vi "fpgaLED.vi"(7 "FPGA I/O In":refnum<k21>="IO Module\\D0 0", 8 "Testpulse Time Delay (20 ns ticks)":u32=15, 9 "Testpulse Separation (20 ns ticks)":u32=500, 10 "Testpulse duration (20 ns ticks)":u32=1, 11 "Testpulser On/Off":bool) -> (0 "Total number of pulses sent":u64, 3 "Is Test Pulse?":bool)   [LabVIEW 2012]
uses:
  <vilib>/rvi/eio/common/nirviEmuTemplateMethod_errors.vi
  <vilib>/eio/EIONode/EIONode.xnode
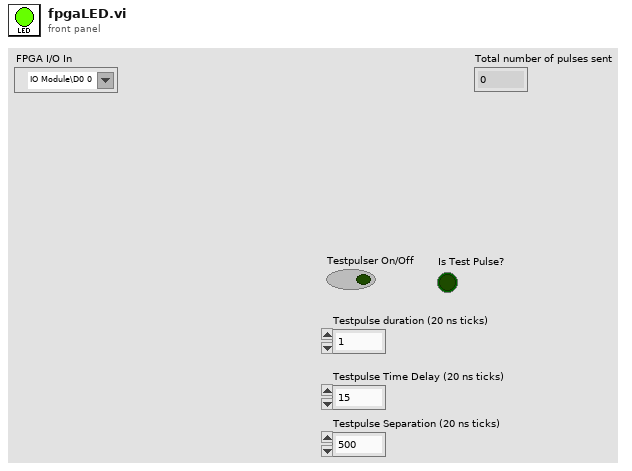
[diagram p1: front panel]
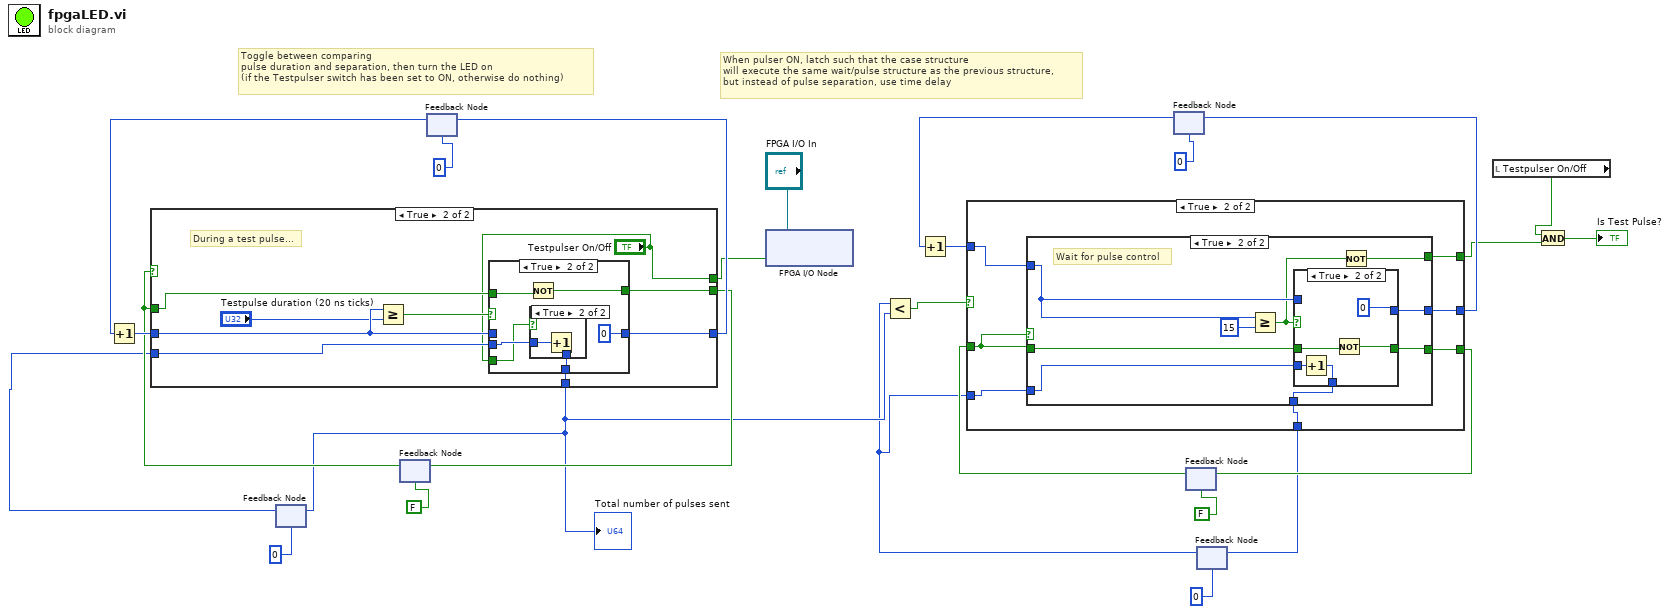
[diagram p0: block diagram]
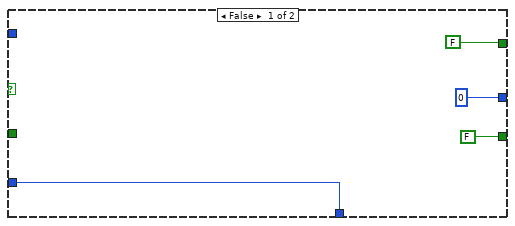
[diagram p2: hidden frame]
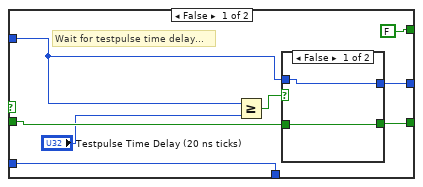
[diagram p3: hidden frame]
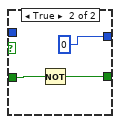
[diagram p4: hidden frame]
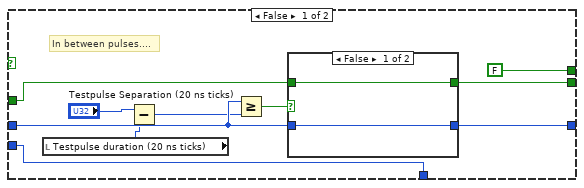
[diagram p6: hidden frame]
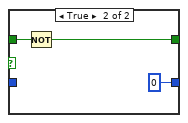
[diagram p7: hidden frame]
diagram:
  # "Toggle between comparing \npulse duration and separation, then turn the LED on\n(if the Testpulser switch has been set to ON, otherwise do nothing)"
  # "When pulser ON, latch such that the case structure\nwill execute the same wait/pulse structure as the previous structure, \nbut instead of pulse separation, use time delay"
  n1 = feedback #1(u64 0) -> (w9:u64)
  n2 = feedback #2(FALSE) -> (w21:bool)
  n3 = feedback #3(u32 0) -> (w24:u32)
  n4 = Increment(x=w24) -> (x+1=w26:u32)
  n5 = case shown="True" w21 {
    tunnel: w26 -> [w33 w48]
    tunnel: [w36 w49] -> w23
    tunnel: [w35 w50] -> w13
    tunnel: [FALSE ("IO Module\\D0 0") "Testpulser On/Off"] -> w12
    tunnel: w21 -> [w31 w45]
    tunnel: w9 -> [w30 w44]
    tunnel: [w30 w43] -> w7
    frame False {
      # "In between pulses...."
      n6 = local read "Testpulse duration (20 ns ticks)"() -> (w27:u32)
      n7 = Subtract(x="Testpulse Separation (20 ns ticks)", y=w27) -> (x-y=w28:u32)
      n8 = Greater Or Equal?(x=w33, y=w28) -> (x >= y?=w32:bool)
      n9 = case shown="False" w32 {
        tunnel: [w38 u32 0] -> w36
        tunnel: w33 -> [w38 _]
        tunnel: [w37 w40] -> w35
        tunnel: w31 -> [w37 w39]
        frame False {
        }
        frame True {
          n10 = Not(x=w39) -> (.not. x?=w40:bool)
        }
      }
    }
    frame True {
      # "During a test pulse..."
      n11 = Greater Or Equal?(x=w48, y="Testpulse duration (20 ns ticks)") -> (x >= y?=w47:bool)
      n12 = case shown="True" w47 {
        tunnel: w48 -> [w53 _]
        tunnel: [w52 w59] -> w50
        tunnel: [w53 u32 0] -> w49
        tunnel: w45 -> [w52 w57]
        tunnel: w44 -> [w51 w56]
        tunnel: [w51 w55] -> w43
        tunnel: "Testpulser On/Off" -> [_ w54]
        frame False {
        }
        frame True {
          n13 = Not(x=w57) -> (.not. x?=w59:bool)
          n14 = case shown="True" w54 {
            tunnel: w56 -> [w60 w62]
            tunnel: [w60 w61] -> w55
            frame False {
            }
            frame True {
              n15 = Increment(x=w62) -> (x+1=w61:u64)
            }
          }
        }
      }
    }
  }
  "Total number of pulses sent" <- w7
  n16 = feedback-in #1(w7) -> ()
  n17 = feedback-in #2(w13) -> ()
  n18 = feedback-in #3(w23) -> ()
  n19 = xnode "FPGA I/O Node"("I/O Item"=w12, "FPGA I/O In"="FPGA I/O In") -> ()  [unwired: 1 out]
  n20 = feedback #4(u32 0) -> (w19:u32)
  n21 = Increment(x=w19) -> (x+1=w18:u32)
  n22 = feedback #5(FALSE) -> (w15:bool)
  n23 = feedback #6(u64 0) -> (w5:u64)
  n24 = Less?(x=w5, y=w7) -> (x < y?=w8:bool)
  n25 = case shown="True" w8 {
    tunnel: [FALSE w70] -> w2
    tunnel: w18 -> [_ w71]
    tunnel: [u32 0 w69] -> w17
    tunnel: w15 -> [_ w73]
    tunnel: [FALSE w72] -> w14
    tunnel: w5 -> [w63 w68]
    tunnel: [w63 w67] -> w4
    frame False {
    }
    frame True {
      n26 = case shown="True" w73 {
        tunnel: w73 -> [w80 w94]
        tunnel: [w79 w93] -> w72
        tunnel: w71 -> [w76 w95]
        tunnel: [FALSE w90] -> w70
        tunnel: [w77 w92] -> w69
        tunnel: w68 -> [w74 w88]
        tunnel: [w74 w87] -> w67
        frame False {
          # "Wait for testpulse time delay..."
          n27 = Greater Or Equal?(x=w76, y="Testpulse Time Delay (20 ns ticks)") -> (x >= y?=w81:bool)
          n28 = case shown="False" w81 {
            tunnel: w80 -> [w83 w86]
            tunnel: [w83 w85] -> w79
            tunnel: [w82 u32 0] -> w77
            tunnel: w76 -> [w82 _]
            frame False {
            }
            frame True {
              n29 = Not(x=w86) -> (.not. x?=w85:bool)
            }
          }
        }
        frame True {
          # "Wait for pulse control"
          n30 = Greater Or Equal?(x=w95, y=u32 15) -> (x >= y?=w89:bool)
          n31 = case shown="True" w89 {
            tunnel: w95 -> [w97 _]
            tunnel: w94 -> [w98 w102]
            tunnel: [w98 w101] -> w93
            tunnel: [w97 u32 0] -> w92
            tunnel: w88 -> [w96 w100]
            tunnel: [w96 w99] -> w87
            frame False {
            }
            frame True {
              n32 = Increment(x=w100) -> (x+1=w99:u64)
              n33 = Not(x=w102) -> (.not. x?=w101:bool)
            }
          }
          n34 = Not(x=w89) -> (.not. x?=w90:bool)
        }
      }
    }
  }
  n35 = feedback-in #4(w17) -> ()
  n36 = feedback-in #5(w14) -> ()
  n37 = feedback-in #6(w4) -> ()
  n38 = local read "Testpulser On/Off"() -> (w1:bool)
  n39 = And(x=w1, y=w2) -> (x .and. y?=→"Is Test Pulse?":bool)
